vi "Signal Params Calculation.vi"(8 "error in":errorcluster, 11 "Signal":dbl[](array[numeric])) -> (0 "error out":errorcluster, 3 "Signal Parameters":T1)   [LabVIEW 2021]
uses:
  Typedefs/Signal Parameters.ctl
  <vilib>/Analysis/5stat.llb/RMS (DBL).vi
  <vilib>/measure/matone.llb/Extract Single Tone Information 1 Chan.vi
  <vilib>/Analysis/NI_AALPro.lvlib
  <vilib>/measure/NI_MAPro.lvlib
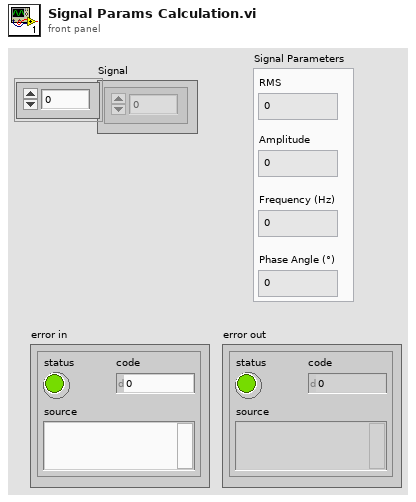
[diagram p1: front panel]
types:
  T1 = typedef "Signal Parameters.ctl" = cluster{"RMS":dbl, "Amplitude":dbl, "Frequency (Hz)":dbl, "Phase Angle (°)":dbl}
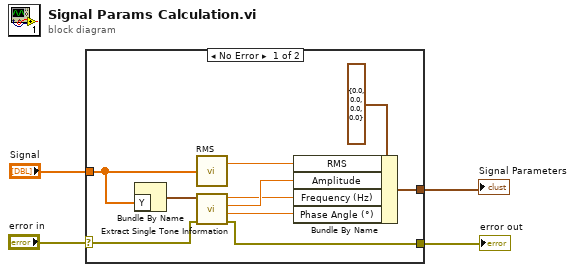
[diagram p0: block diagram]
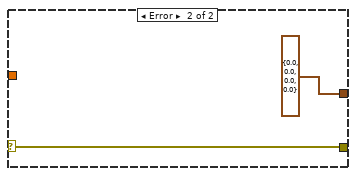
[diagram p2: hidden frame]
diagram:
  n1 = case shown="No Error" "error in" {
    selector: "error in" -> [w6 w16]
    tunnel: [w10 T1 {"RMS"=0.0, "Amplitude"=0.0, "Frequency (Hz)"=0.0, "Phase Angle (°)"=0.0} ("Phase 1 Voltage")] -> w4
    tunnel: "Signal" -> [w7 _]
    tunnel: [w5 w16] -> w1
    frame No Error {
      n2 = Bundle By Name("Y"=w7) -> (w11:waveform(dbl))  [unwired: 1 in]
      n3 = call-poly <vilib>:"RMS.vi"("X"=w7) -> ("rms value"=w9:dbl)  [unwired: 1 out]
      n4 = call-poly <vilib>:"Extract Single Tone Information.vi"("error in (no error)"=w6, "time signal in"=w11) -> ("error out"=w5:errorcluster, "detected phase (deg)"=w14:dbl, "detected amplitude"=w13:dbl, "detected frequency"=w12:dbl)  [unwired: 4 in, 2 out]
      n5 = Bundle By Name(cluster=T1 {"RMS"=0.0, "Amplitude"=0.0, "Frequency (Hz)"=0.0, "Phase Angle (°)"=0.0} ("Phase 1 Voltage"), "RMS"=w9, "Amplitude"=w13, "Frequency (Hz)"=w12, "Phase Angle (°)"=w14) -> (w10:T1)
    }
    frame Error {
    }
  }
  "Signal Parameters" <- w4
  "error out" <- w1
